vi "Find First Number.vi"(11 "String in":string) -> (3 "first number string":string)   [LabVIEW 2022 SP3]
uses:
  <vilib>/regexp/Match Regular Expression.xnode
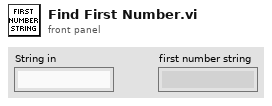
[diagram p1: front panel]
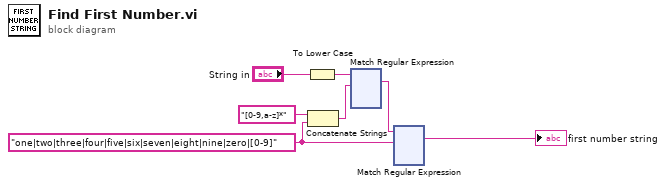
[diagram p0: block diagram]
diagram:
  w2 = "one|two|three|four|five|six|seven|eight|nine|zero|[0-9]" ("format string")
  n1 = To Lower Case(string="String in") -> (all lower case string=w6:string)
  n2 = Concatenate Strings("[0-9,a-z]*" ("format string"), w2) -> (w3:string)
  n3 = xnode "Match Regular Expression"("input string"=w6, "regular expression"=w3) -> ("whole match"=w5:string)  [unwired: 4 in, 4 out]
  n4 = xnode "Match Regular Expression"("input string"=w5, "regular expression"=w2) -> ("whole match"=→"first number string":string)  [unwired: 4 in, 4 out]
